vi "计算.vi"(8 "error in (no error)":errorcluster caption="错误输入（无错误）", 11 "平方和类 输入":refnum<class "平方和类.lvclass"> caption="DNL_LabVIEW Object in") -> (0 "error out":errorcluster caption="错误输出", 2 "结果":dbl, 3 "平方和类 输出":refnum<class "平方和类.lvclass"> caption="DNL_LabVIEW Object out")   [LabVIEW 2013, in "平方和类.lvclass"]
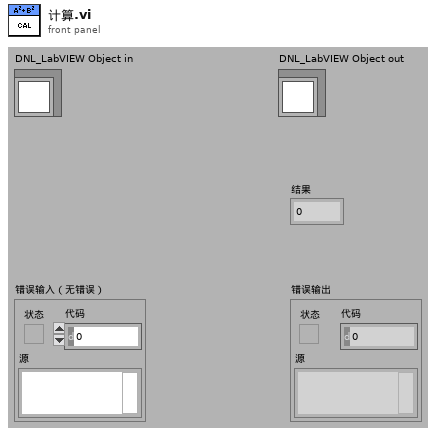
[diagram p1: front panel]
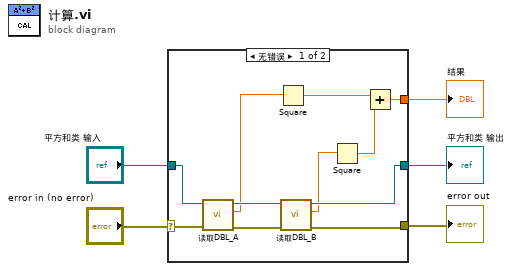
[diagram p0: block diagram]
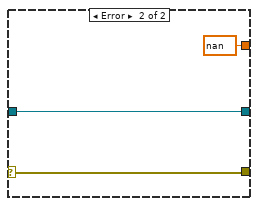
[diagram p2: hidden frame]
diagram:
  n1 = case shown="无错误" "error in (no error)" {
    selector: "error in (no error)" -> [w16 w19]
    tunnel: [w14 w19] -> w4
    tunnel: [w11 w18] -> w2
    tunnel: "平方和类 输入" -> [w13 w18]
    tunnel: [w6 nan] -> w1
    frame No Error {
      n2 = call "读取DBL_A.vi"("error in (no error)"=w16, "运算类输入"=w13) -> ("error out"=w15:errorcluster, "DBL_A"=w10:dbl, "运算类输出"=w12:refnum<class "平方和类.lvclass">)  [unwired: 7 in]
      n3 = Square(x=w10) -> (x^2=w8:dbl)
      n4 = call "读取DBL_B.vi"("error in (no error)"=w15, "运算类输入"=w12) -> ("error out"=w14:errorcluster, "DBL_B"=w9:dbl, "运算类输出"=w11:refnum<class "平方和类.lvclass">)  [unwired: 7 in]
      n5 = Square(x=w9) -> (x^2=w7:dbl)
      n6 = Add(x=w8, y=w7) -> (x+y=w6:dbl)
    }
    frame Error {
    }
  }
  "error out" <- w4
  "平方和类 输出" <- w2
  "结果" <- w1
